vi "FP Server Get Data.vi"(6 "Values and Position":refnum<vi>[](array[refnum]), 8 "error in (no error)":errorcluster, 9 "Message":string="GetData", 10 "Connection ID":u64, 11 "Page":string) -> (0 "error out":errorcluster)   [LabVIEW 2017, in "Front Panel Publisher.lvlib" / "Front Panel Manager.lvclass"]
uses:
  Front Panel Manager.lvclass
  Protected/FP Server Message.ctl
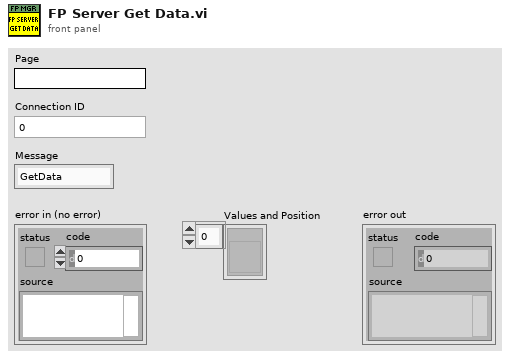
[diagram p1: front panel]
types:
  T1 = typedef "Front Panel Publisher.lvlib/Front Panel Manager.lvclass/FP Server Message.ctl" = cluster{"Message":string, "Page":string, "Data":string[][], "Connection ID":u64, "Values and Position":refnum<vi>[]}
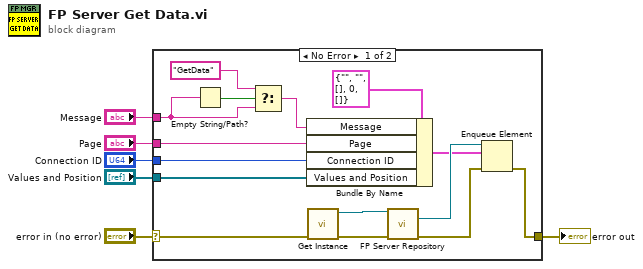
[diagram p0: block diagram]
diagram:
  n1 = case shown="No Error" "error in (no error)" {
    selector: "error in (no error)" -> [w18 w22]
    tunnel: [w13 w22] -> w5
    tunnel: "Page" -> [w14 _]
    tunnel: "Connection ID" -> [w12 _]
    tunnel: "Message" -> [w10 _]
    tunnel: "Values and Position" -> [w7 _]
    frame No Error {
      n2 = Empty String/Path?(string/path=w10) -> (empty?=w11:bool)
      n3 = Select(t="GetData", s=w11, f=w10) -> (s? t:f=w8:string)
      n4 = Bundle By Name(cluster=T1 {"Message"="", "Page"="", "Data"=[], "Connection ID"=0, "Values and Position"=[]} ("element"), "Message"=w8, "Page"=w14, "Connection ID"=w12, "Values and Position"=w7) -> (w15:T1)
      n5 = call "Get Instance.vi"("error in (no error)"=w18) -> ("error out"=w17:errorcluster, "FP Manager Out"=w19:refnum<class "Front Panel Manager.lvclass">)  [unwired: 6 in, 3 out]
      n6 = call "FP Server Repository.vi"("FP Management In"=w19, "error in (no error)"=w17) -> ("ToProcessQueue"=w16:refnum<queue>, "error out"=w20:errorcluster)  [unwired: 7 in, 5 out]
      n7 = Enqueue Element(queue=w16, element=w15, error in (no error)=w20) -> (error out=w13:errorcluster)  [unwired: 1 in, 2 out]
    }
    frame Error {
    }
  }
  "error out" <- w5
